vi "Apply.vi"(8 "error in (no error)":errorcluster, 11 "IConfigurable in":refnum<class "IConfigurable.lvclass">) -> (0 "error out":errorcluster, 3 "IConfigurable out":refnum<class "IConfigurable.lvclass">)   [LabVIEW 2023, in "IConfigurable.lvclass"]
uses:
  IConfigurable.lvclass
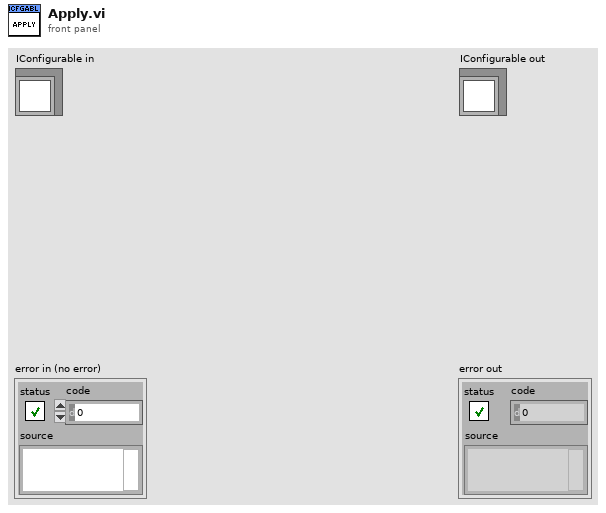
[diagram p1: front panel]
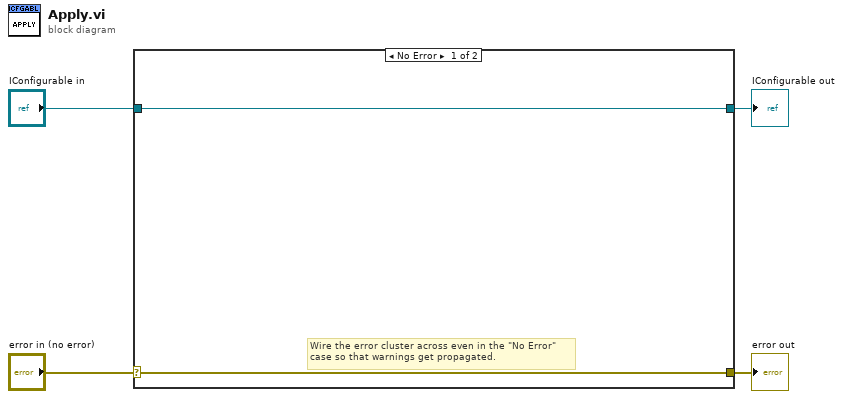
[diagram p0: block diagram]
diagram:
  n1 = case shown="No Error" "error in (no error)" {
    selector: "error in (no error)" -> [w5 w8]
    tunnel: [w5 w8] -> w3
    tunnel: [w6 w7] -> w1
    tunnel: "IConfigurable in" -> [w6 w7]
    frame No Error {
      # "Wire the error cluster across even in the \"No Error\"\ncase so that warnings get propagated."
    }
    frame Error {
    }
  }
  "error out" <- w3
  "IConfigurable out" <- w1
